vi "LeCroy.Read Single Waveform.vi"(5 "Source":u16(ring) items=["Channel 1", "Channel 2", "Channel 3", "Channel 4", "Memory 1", "Memory 2", "Memory 3", "Memory 4", "Function 1", "Function 2", "Function 3", "Function 4", "Function 5", "Function 6", "Function 7", "Function 8", "Other"], 8 "Error In":errorcluster, 11 "LeCroy.Session in":T1) -> (0 "Error Out":errorcluster, 2 "Waveform Data":waveform(dbl), 3 "LeCroy.Session out":T1)   [LabVIEW 2018]
uses:
  typedefs/LeCroy.Session.ctl
  Driver/lecroy_wave_series/LeCroy Wave Series/Public/Data/Read Single Waveform.vi
  Driver/lecroy_wave_series/LeCroy Wave Series/LeCroy Wave Series.lvlib
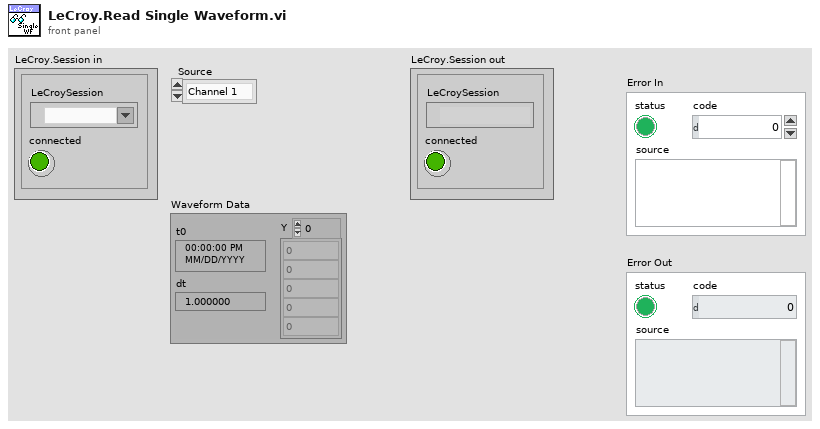
[diagram p1: front panel]
types:
  T1 = typedef "LeCroy.Session.ctl" = cluster{"LeCroySession":refnum<visa-resource-name>, "connected":bool}
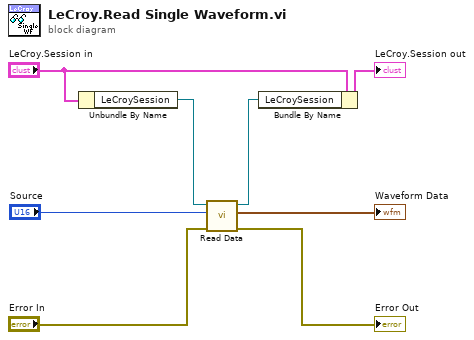
[diagram p0: block diagram]
diagram:
  n1 = Unbundle By Name("LeCroy.Session in") -> ("LeCroySession"=w6:refnum<visa-resource-name>)
  n2 = call-poly "Read Data.vi"("error in (no error)"="Error In", "Source (0: Channel 1)"="Source", "VISA resource name"=w6) -> ("error out"=→"Error Out":errorcluster, "Waveform Data"=→"Waveform Data":waveform(dbl), "VISA resource name out"=w5:refnum<visa-resource-name>)  [unwired: 6 in]
  n3 = Bundle By Name(cluster="LeCroy.Session in", "LeCroySession"=w5) -> (→"LeCroy.Session out":T1)
